vi "reset.vi"(8 "error in (no error)":errorcluster, 11 "channel":u16 format="%x") -> (0 "error out":errorcluster)   [LabVIEW 2024, in "atsj peakcan basic.lvlib"]
doc: "Resets the receive and transmit queues of a PCAN <b>channel</b>."
uses:
  atsj peakcan basic.lvlib
  support/x64/PCANBasic.dll
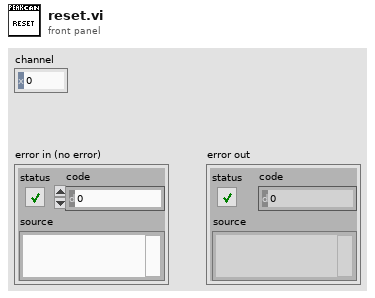
[diagram p1: front panel]
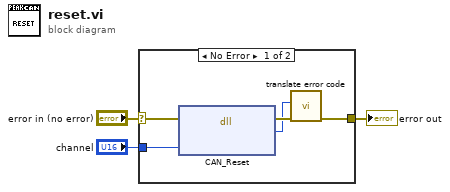
[diagram p0: block diagram]
diagram:
  n1 = case shown="No Error" "error in (no error)" {
    selector: "error in (no error)" -> [w7 w9]
    tunnel: [w4 w9] -> w1
    tunnel: "channel" -> [w8 _]
    frame No Error {
      n2 = dll-call lib="C:/atsj/plateau/atsj-peakcan-basic-for-labview/src/support/x64/PCANBasic.dll" fn="CAN_Reset" ("reset")(error in=w7, "Channel"=w8) -> (error out=w6:errorcluster, "Status"=w5:u32)  [unwired: 3 in, 1 out]
      n3 = call "translate error code.vi"("error in (no error)"=w6, "error code"=w5) -> ("error out"=w4:errorcluster)  [unwired: 9 in]
    }
    frame Error {
    }
  }
  "error out" <- w1
